vi "getSubData_MagSpec.vi"(7 "index":i32, 9 "image in":T1, 10 "SubscriberCluster":T2, 11 "timeout (s)":dbl=3000.0) -> (3 "image out":T1)   [LabVIEW 2013]
uses:
  shared/SubscriberCluster_TypDEf.ctl
  Interface/Sandbox/GUI_Template/GUI_master/tcp_new_data_event.ctl
  Interface/Sandbox/GUI_Template/GUI_master/tcp new data cluster.ctl
  <vilib>/vision/Image Controls.llb/IMAQ Image.ctl
  <userlib>/_OpenG.lib/array/array.llb/Remove Duplicates from 1D Array (String)__ogtk.vi
panel:
  out "Device name":string
  out "timed out?":bool
  out "element":string[][](array[string])
  out "Numeric":i32
  out "timeout":bool
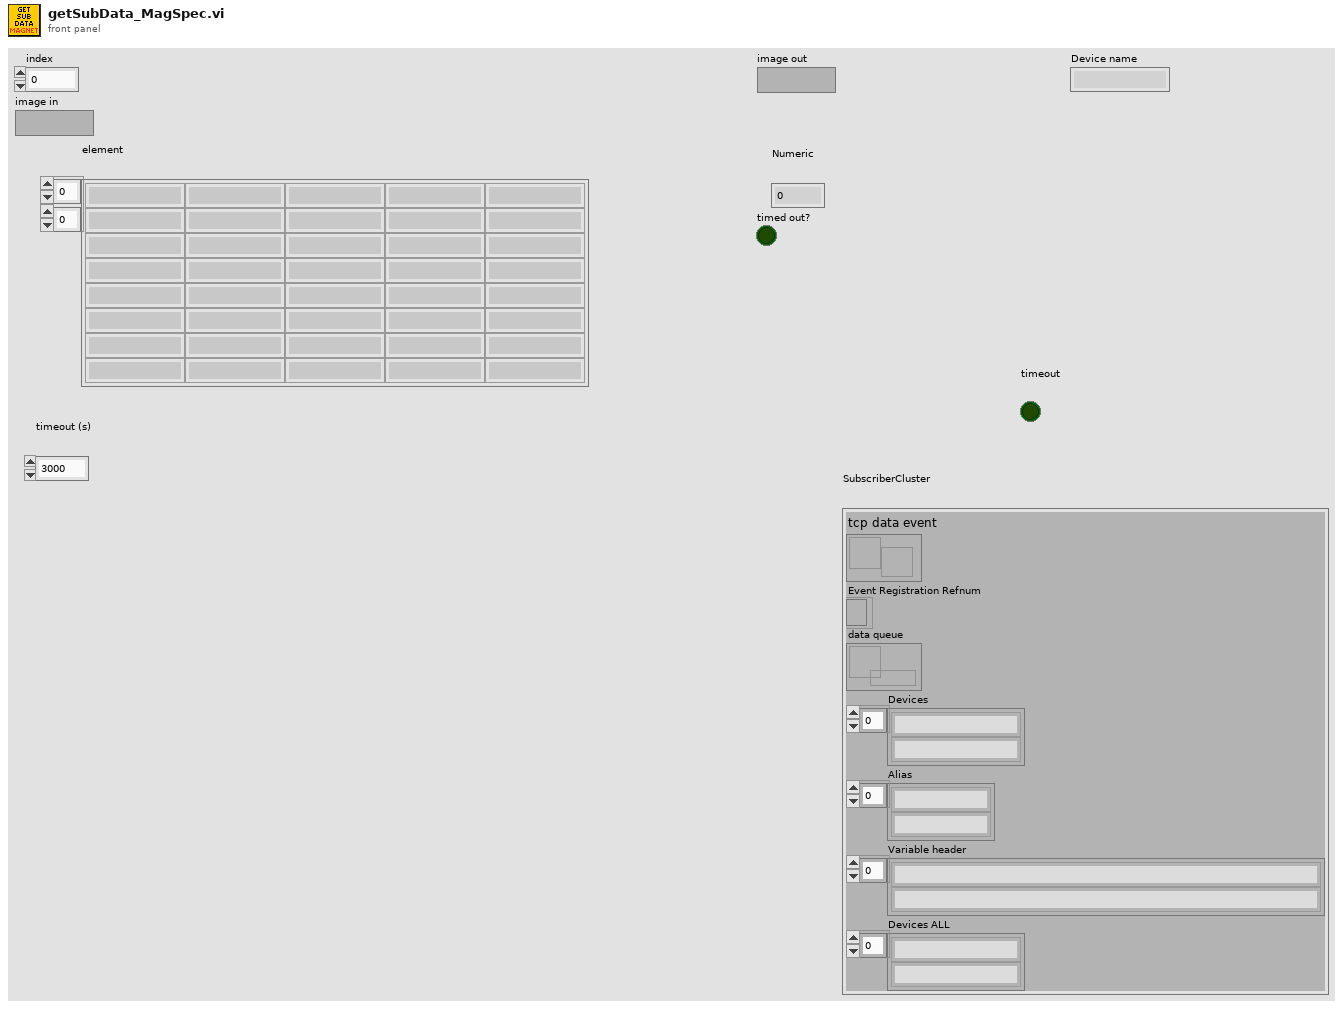
[diagram p1: front panel]
types:
  T1 = typedef "IMAQ Image.ctl" = refnum<image>
  T2 = typedef "SubscriberCluster_TypDEf.ctl" = cluster{"tcp data event":T3, "Event Registration Refnum":refnum<event-registration>, "data queue":refnum<queue>, "Devices":string[], "Alias":string[], "Variable header":string[], "Devices ALL":string[]}
  T3 = typedef "tcp_new_data_event.ctl" = refnum<user-event>
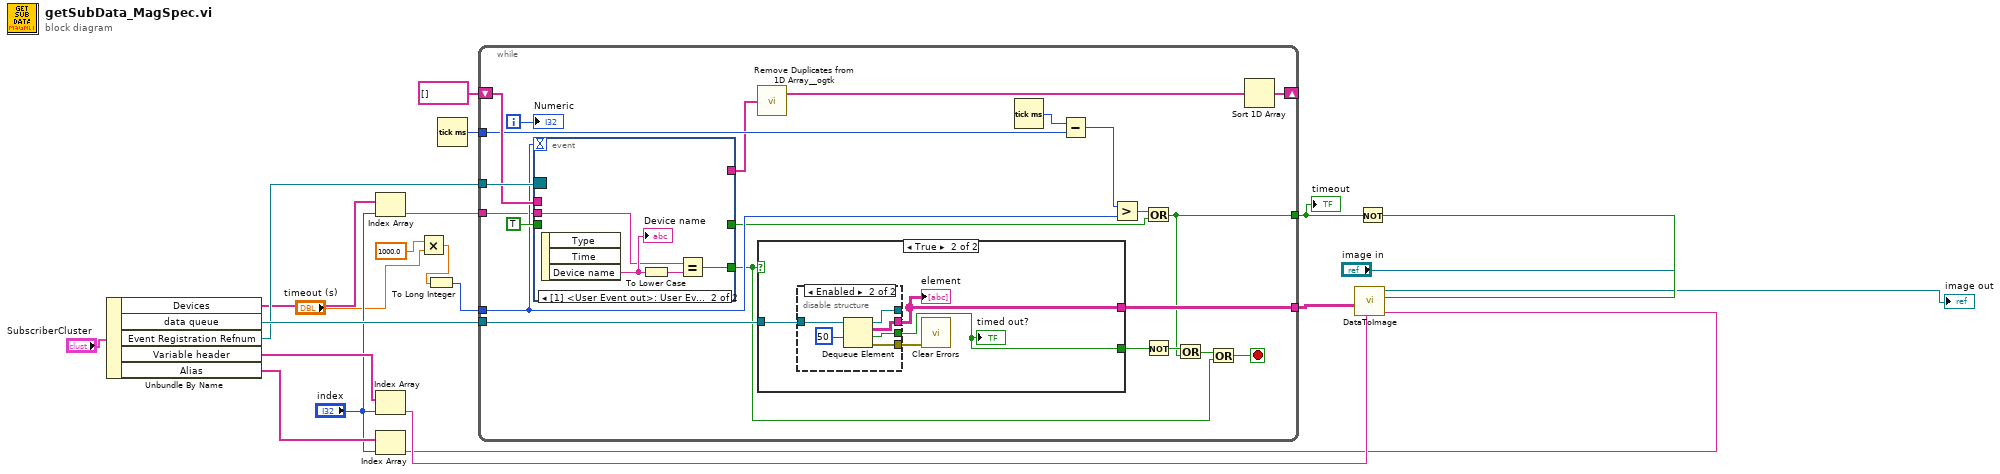
[diagram p0: block diagram]
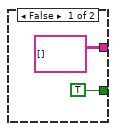
[diagram p2: hidden frame]
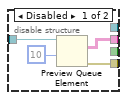
[diagram p3: hidden frame]
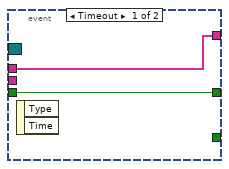
[diagram p4: hidden frame]
diagram:
  n1 = Unbundle By Name("SubscriberCluster") -> ("Devices"=w13:string[], "data queue"=w19:refnum<queue>, "Event Registration Refnum"=w18:refnum<event-registration>, "Variable header"=w11:string[], "Alias"=w9:string[])
  n2 = Index Array(array=w13, index="index") -> (element=w12:string)
  n3 = Index Array(array=w11, index="index") -> (element=w10:string)
  n4 = Index Array(array=w9, index="index") -> (element=w7:string)
  n5 = Multiply(x=1000.0, y="timeout (s)") -> (x*y=w4:dbl)
  n6 = To Long Integer(number=w4) -> (32bit integer=w3:i32)
  n7 = Tick Count (ms)() -> (millisecond timer value=w16:u32)
  n8 = while {
    tunnel: w18 -> [w43]
    tunnel: w19 -> [w35]
    tunnel: [w34] -> w17
    shift-right: [w32] -> _
    shift-left: string[] [] -> [w41]
    tunnel: w3 -> [w38]
    tunnel: [w27] -> w15
    tunnel: w16 -> [w40]
    tunnel: w12 -> [w26]
    i -> [w33]
    stop <- w22 stop-if-true
    n9 = event shown="[1] <User Event out>: User Event" {
      selector: w43 -> [_ _]
      dyn-events: _ -> [_ _]
      timeout: w38 -> [_ _]
      tunnel: [w61 _] -> w25
      tunnel: TRUE -> [w61 _]
      tunnel: [w60 _] -> w31
      tunnel: w41 -> [w60 _]
      tunnel: w26 -> [_ w63]
      tunnel: [_ w62] -> w23
      event Timeout {
        n10 = event-data() -> ()  [unwired: 1 in, 2 out]
      }
      event User Event {
        n11 = event-data() -> ("Device name"=w65:string)  [unwired: 1 in, 2 out]
        "Device name" <- w65
        n12 = To Lower Case(string=w65) -> (all lower case string=w64:string)
        n13 = Equal?(x=w63, y=w64) -> (x = y?=w62:bool)
      }
    }
    n14 = call-poly <userlib>:"Remove Duplicates from 1D Array__ogtk.vi"("Input Array"=w31) -> ("Output Array"=w30:string[])  [unwired: 1 out]
    n15 = case shown="True" w23 {
      tunnel: w35 -> [_ w49]
      tunnel: [string[][] [] ("Data in") w47] -> w34
      tunnel: [TRUE ("timed out?") w46] -> w29
      frame False {
      }
      frame True {
        n16 = disable-structure shown="Enabled" {
          disable-tunnel: w49 -> [w52 w59]
          disable-tunnel: [w51 w58] -> w47
          disable-tunnel: [w50 w57] -> w48
          disable-tunnel: [_ w55] -> _
          disable-tunnel: [_ w54] -> w46
          frame Disabled {
            n17 = Preview Queue Element(queue=w52, timeout in ms (-1)=10) -> (element=w51:string[][], error out=w50:errorcluster)  [unwired: 1 in, 2 out]
          }
          frame Enabled {
            n18 = Dequeue Element(queue=w59, timeout in ms (-1)=50) -> (queue out=w55:refnum<queue>, element=w58:string[][], timed out?=w54:bool, error out=w57:errorcluster)  [unwired: 1 in]
          }
        }
        "element" <- w47
        "timed out?" <- w46
        n19 = call <vilib>:"Clear Errors.vi"("error in (no error)"=w48) -> ()  [unwired: 6 in, 1 out]
      }
    }
    n20 = Tick Count (ms)() -> (millisecond timer value=w36:u32)
    n21 = Subtract(x=w36, y=w40) -> (x-y=w39:u32)
    n22 = Greater?(x=w39, y=w38) -> (0:w37:bool)
    n23 = Or(x=w37, y=w25) -> (x .or. y?=w27:bool)
    n24 = Not(x=w29) -> (.not. x?=w28:bool)
    n25 = Or(x=w28, y=w27) -> (x .or. y?=w24:bool)
    n26 = Or(x=w24, y=w23) -> (x .or. y?=w22:bool)
    n27 = Sort 1D Array(array=w30) -> (sorted array=w32:string[])
    "Numeric" <- w33
  }
  "timeout" <- w15
  n28 = Not(x=w15) -> (.not. x?=w14:bool)
  n29 = call "DataToImage.vi"("String"=w10, "userID"=w7, "Data in"=w17, "Boolean"=w14, "Refnum in"="image in") -> ("Refnum out"=→"image out":T1)  [unwired: 6 in]
